vi "emi_DNU 1D array of Variant to Variant with Array.vi"(0 "Array Type":variant, 5 "1D Array of Variant":variant[](array[variant]), 9 "Single Element TD":i16[](array[numeric]), 11 "error in":errorcluster) -> (4 "Array":variant, 15 "error out":errorcluster)   [LabVIEW 2010]
doc: "Combine an Variant with an array for Type, with a TD defenition of the contained element, and an array of variants with the same contained elements.\n\nFIKK IKKE TIL Å BRUKE DENNE I SKRIVING/LESING AV INI FILE. TROR DEN GJØR DET DEN SKAL; MEN AT DET ER BRUKEN SOM ER FEIL:\n\nThis could probably be done a bit simpler, but...\n\nIntended for use in ini file reading together with \"Variant With Array to 1D array of Variant.vi\""
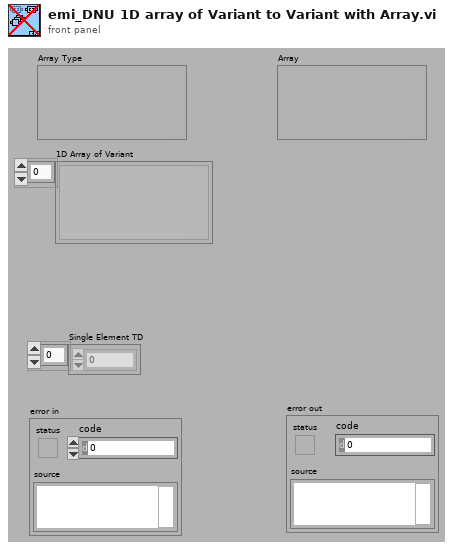
[diagram p1: front panel]
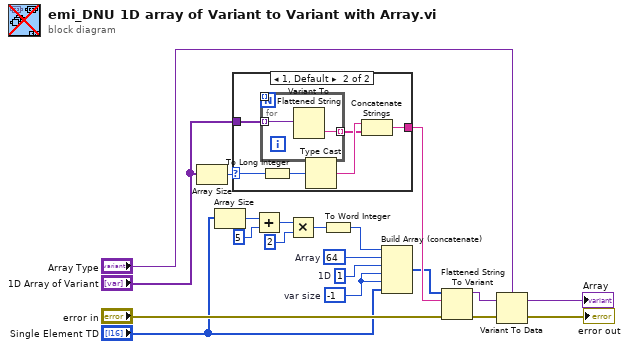
[diagram p0: block diagram]
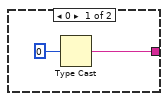
[diagram p2: hidden frame]
diagram:
  w7 = i16 -1  # var size
  w6 = i16 1  # 1D
  w5 = i16 64  # Array
  n1 = Array Size(array="1D Array of Variant") -> (size(s)=w12:i32)
  n2 = Array Size(array="Single Element TD") -> (size(s)=w1:i32)
  n3 = case shown="1, Default" w12 {
    selector: w12 -> [_ w27]
    tunnel: "1D Array of Variant" -> [_ w28]
    tunnel: [w22 w23] -> w14
    frame 0 {
      n4 = Type Cast(x=0) -> (*(type *) &x=w22:string)  [unwired: 1 in]
    }
    frame 1, Default {
      n5 = for {
        N -> [w29]
        tunnel: w28 -> [w31] mode=indexing
        tunnel: [w30] -> w24 mode=indexing
        tunnel: [w29] -> _ mode=indexing
        n6 = Variant To Flattened String(Variant=w31) -> (data string=w30:string)  [unwired: 1 out]
      }
      n7 = To Long Integer(number=w27) -> (32bit integer=w26:i32)
      n8 = Type Cast(x=w26) -> (*(type *) &x=w25:string)  [unwired: 1 in]
      n9 = Concatenate Strings(w25, w24) -> (w23:string)
    }
  }
  n10 = Add(x=w1, y=5) -> (x+y=w3:i32)
  n11 = Multiply(x=w3, y=2) -> (x*y=w8:i32)
  n12 = To Word Integer(number=w8) -> (16bit integer=w9:i16)
  n13 = Build Array (concatenate)(w9, w5, w6, w7, w7, "Single Element TD") -> (w10:i16[])
  n14 = Flattened String To Variant(4:"error in", 6:w14, 7:w10) -> (0:w16:errorcluster, 3:w18:variant)
  n15 = Variant To Data(error in=w16, Variant=w18, type="Array Type") -> (error out=→"error out":errorcluster, data=→"Array":variant)
